vi "Graphics-Sort XY Graph (scalar).vi"(7 "graph":cluster{"x":dbl[], "y":dbl[]}) -> (8 "sorted graph":cluster{"x":dbl[], "y":dbl[]})   [LabVIEW 2020]
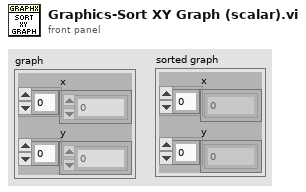
[diagram p1: front panel]
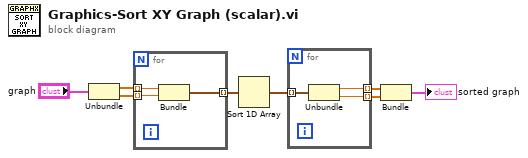
[diagram p0: block diagram]
diagram:
  n1 = Unbundle("graph") -> ("x"=w6:dbl[], "y"=w5:dbl[])
  n2 = for {
    tunnel: w6 -> [w11] mode=indexing
    tunnel: [w10] -> w8 mode=indexing
    tunnel: w5 -> [w9] mode=indexing
    n3 = Bundle("Numeric"=w11, "Numeric"=w9) -> (w10:cluster{"Numeric":dbl, "Numeric":dbl})  [unwired: 1 in]
  }
  n4 = Sort 1D Array(array=w8) -> (sorted array=w4:cluster{"Numeric":dbl, "Numeric":dbl}[])
  n5 = for {
    tunnel: w4 -> [w14] mode=indexing
    tunnel: [w13] -> w3 mode=indexing
    tunnel: [w12] -> w2 mode=indexing
    n6 = Unbundle(w14) -> ("Numeric"=w13:dbl, "Numeric"=w12:dbl)
  }
  n7 = Bundle(w3, w2) -> (→"sorted graph":cluster{dbl[], dbl[]})  [unwired: 1 in]
